vi "pp3_DAQ_AudioTriggerPlay.vi"(0 "Daq config In":T6={"Sound AO"="Dev2/ao0", "Shock intesity AO"="Dev1/ao1", "Code_LED DO"="Dev1/port1:2", "Switch DI"="Dev1/port0/line0:1", "Webcam"="cam0", "Sound AO task"="", "Sound card task"=0, "Shock intensity AO task"="", "Code_LED DO task"="", "Switch DI task"="", "AO <=> Sound card"=FALSE, "Sound card"=0, "sample rate"=8000.0, "Variable shock"=FALSE, "Webcam on"=FALSE, "Tone gate PFI"="/Dev1/PFI1", "Waveform memo"={"t0"=timestamp(0 s since 1904-01-01), "dt"=1.0, "Y"=[]}, "First time"=FALSE} {"sample rate" min=8000.0; "Sound card task" format="%.0x"}, 5 "State In":T1={"Curr  tr"=0, "Curr (ms)"=0, "Cum (ms)"=0, "Run loop diff"=0, "Tone countdown (ms)"=0, "Countdown (ms)"=0, "Curr State"=enum."0 NULL", "Prev State"=enum."1 Habituation", "Rw"=FALSE, "Sw"=FALSE, "Tone\nGate"=FALSE, "Punish"=FALSE, "Current DAQ DO Int"=0, "Current Loaded Trial"={"Trial Type Number"=1, "Trial Type"=enum."GO", "Trial Weight"=100, "Shock (mA)"=0.3, "Duration (ms)"=0.25, "Sound Type"=enum."04 FM Sweep", "Stim P1"=4000.0, "Stim P2"=0.0, "Stim P3"=0.0, "Stim P4"=2000.0, "DAQ Amplitude (V)"=0.25}, "Next Trial (for display purposes)"={"Trial Type Number"=1, "Trial Type"=enum."GO", "Trial Weight"=100, "Shock (mA)"=0.3, "Duration (ms)"=0.25, "Sound Type"=enum."04 FM Sweep", "Stim P1"=4000.0, "Stim P2"=0.0, "Stim P3"=0.0, "Stim P4"=2000.0, "DAQ Amplitude (V)"=0.25}, "Total trials memo"=0, "State start cum memo (ms)"=0, "Last dur jump time memo (ms)"=0, "Last dur shock time memo (ms)"=0, "Tone repeat memo (ms)"=0, "Webcam on"=FALSE, "Webcam recording"=FALSE, "State update flag"=FALSE, "Last loaded shock voltage"=0.0, "Vid upd"=enum."0"} {"Current DAQ DO Int" format="%016b"; "Next Trial (for display purposes)"."DAQ Amplitude (V)" min=0.0 max=5.0 format="%_6g"; "Next Trial (for display purposes)"."Shock (mA)" min=-1.0 max=5.0; "Next Trial (for display purposes)"."Trial Weight" step=1; "Next Trial (for display purposes)"."Duration (ms)" min=0.0 max=1.0; "Next Trial (for display purposes)"."Trial Type Number" min=1 max=256 step=1; "Current Loaded Trial"."DAQ Amplitude (V)" min=0.0 max=5.0 format="%_6g"; "Current Loaded Trial"."Shock (mA)" min=-1.0 max=5.0; "Current Loaded Trial"."Trial Weight" step=1; "Current Loaded Trial"."Duration (ms)" min=0.0 max=1.0; "Current Loaded Trial"."Trial Type Number" min=1 max=256 step=1}, 11 "error in (no error)":errorcluster) -> (4 "Daq config Out":T6={"Sound AO"="Dev2/ao0", "Shock intesity AO"="Dev1/ao1", "Code_LED DO"="Dev1/port1:2", "Switch DI"="Dev1/port0/line0:1", "Webcam"="cam0", "Sound AO task"="", "Sound card task"=0, "Shock intensity AO task"="", "Code_LED DO task"="", "Switch DI task"="", "AO <=> Sound card"=FALSE, "Sound card"=0, "sample rate"=8000.0, "Variable shock"=FALSE, "Webcam on"=FALSE, "Tone gate PFI"="/Dev1/PFI1", "Waveform memo"={"t0"=timestamp(0 s since 1904-01-01), "dt"=1.0, "Y"=[]}, "First time"=FALSE} {"sample rate" min=8000.0; "Sound card task" format="%.0x"}, 6 "State Out":T1={"Curr  tr"=0, "Curr (ms)"=0, "Cum (ms)"=0, "Run loop diff"=0, "Tone countdown (ms)"=0, "Countdown (ms)"=0, "Curr State"=enum."0 NULL", "Prev State"=enum."1 Habituation", "Rw"=FALSE, "Sw"=FALSE, "Tone\nGate"=FALSE, "Punish"=FALSE, "Current DAQ DO Int"=0, "Current Loaded Trial"={"Trial Type Number"=1, "Trial Type"=enum."GO", "Trial Weight"=100, "Shock (mA)"=0.3, "Duration (ms)"=0.25, "Sound Type"=enum."04 FM Sweep", "Stim P1"=4000.0, "Stim P2"=0.0, "Stim P3"=0.0, "Stim P4"=2000.0, "DAQ Amplitude (V)"=0.25}, "Next Trial (for display purposes)"={"Trial Type Number"=1, "Trial Type"=enum."GO", "Trial Weight"=100, "Shock (mA)"=0.3, "Duration (ms)"=0.25, "Sound Type"=enum."04 FM Sweep", "Stim P1"=4000.0, "Stim P2"=0.0, "Stim P3"=0.0, "Stim P4"=2000.0, "DAQ Amplitude (V)"=0.25}, "Total trials memo"=0, "State start cum memo (ms)"=0, "Last dur jump time memo (ms)"=0, "Last dur shock time memo (ms)"=0, "Tone repeat memo (ms)"=0, "Webcam on"=FALSE, "Webcam recording"=FALSE, "State update flag"=FALSE, "Last loaded shock voltage"=0.0, "Vid upd"=enum."0"} {"Current DAQ DO Int" format="%016b"; "Next Trial (for display purposes)"."DAQ Amplitude (V)" min=0.0 max=5.0 format="%_6g"; "Next Trial (for display purposes)"."Shock (mA)" min=-1.0 max=5.0; "Next Trial (for display purposes)"."Trial Weight" step=1; "Next Trial (for display purposes)"."Duration (ms)" min=0.0 max=1.0; "Next Trial (for display purposes)"."Trial Type Number" min=1 max=256 step=1; "Current Loaded Trial"."DAQ Amplitude (V)" min=0.0 max=5.0 format="%_6g"; "Current Loaded Trial"."Shock (mA)" min=-1.0 max=5.0; "Current Loaded Trial"."Trial Weight" step=1; "Current Loaded Trial"."Duration (ms)" min=0.0 max=1.0; "Current Loaded Trial"."Trial Type Number" min=1 max=256 step=1}, 15 "error out":errorcluster)   [LabVIEW 2013]
uses:
  pp2_CTL_DaqConfig.ctl
  <vilib>/userdefined/High Color/IMAQdx.ctl
  <vilib>/sound2/lvsound2.llb/Sound Output Task ID.ctl
  pp3_CTL_StateInfo.ctl
  pp3_CTL_State.ctl
  pp3_CTL_Trial.ctl
  pp3_CTL_TrialType.ctl
  labolabo2/waveforms/WFTypes.ctl
  <vilib>/sound2/lvsound2.llb/Sound Output Write (DBL Single).vi
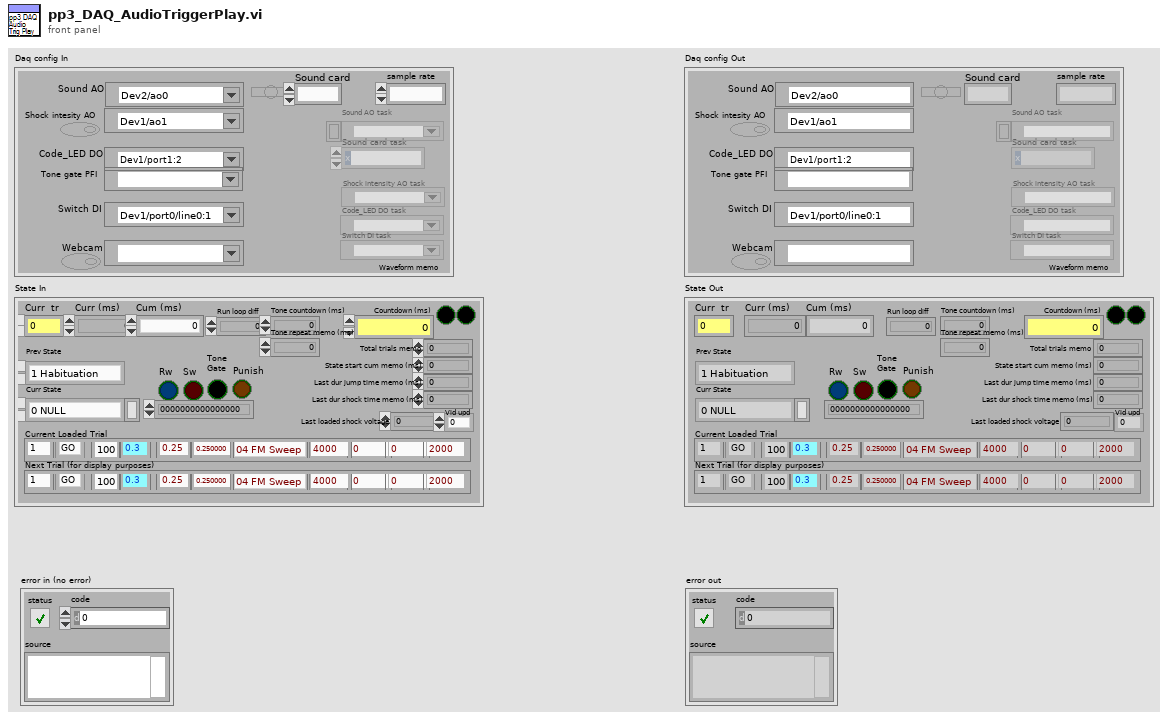
[diagram p1: front panel]
types:
  T1 = typedef "pp3_CTL_StateInfo.ctl" = cluster{"Curr  tr":u16, "Curr (ms)":u32, "Cum (ms)":i64, "Run loop diff":i64, "Tone countdown (ms)":i64, "Countdown (ms)":i64, "Curr State":T2, "Prev State":T2, "Rw":bool, "Sw":bool, "Tone\nGate":bool, "Punish":bool, "Current DAQ DO Int":u16, "Current Loaded Trial":T3, "Next Trial (for display purposes)":T3, "Total trials memo":i64, "State start cum memo (ms)":i64, "Last dur jump time memo (ms)":i64, "Last dur shock time memo (ms)":i64, "Tone repeat memo (ms)":i64, "Webcam on":bool, "Webcam recording":bool, "State update flag":bool, "Last loaded shock voltage":dbl, "Vid upd":enum16{"0", "1", "2", "3", "4", "5", "6", "7", "8", "9"}}
  T2 = typedef "pp3_CTL_State.ctl" = enum8{"0 NULL", "1 Habituation", "2 (Load Trial)", "3 Stay Period", "4 Load Audio/Click Delay", "5 GO Trial", "6 GO Jumped", "7 GO Timeout", "8 NOGO Trial", "9 NOGO Jumped", "10 NOGO Timeout", "11 TEST Trial", "12 TEST Jumped", "13 TEST Timeout", "14 Intertrial Interval", "15 Done"}
  T3 = typedef "pp3_CTL_Trial.ctl" = cluster{"Trial Type Number":i16, "Trial Type":T4, "Trial Weight":u32, "Shock (mA)":dbl, "Duration (ms)":dbl, "Sound Type":T5, "Stim P1":dbl, "Stim P2":dbl, "Stim P3":dbl, "Stim P4":dbl, "DAQ Amplitude (V)":dbl}
  T4 = typedef "pp3_CTL_TrialType.ctl" = enum16{"OFF", "GO", "NOGO", "TEST"}
  T5 = typedef "WFTypes.ctl" = enum16{"00 NULL", "01 DC", "02 Noise", "03 Pure Tone", "04 FM Sweep"}
  T6 = typedef "pp2_CTL_DaqConfig.ctl" = cluster{"Sound AO":tag, "Shock intesity AO":tag, "Code_LED DO":tag, "Switch DI":tag, "Webcam":T7, "Sound AO task":refnum<k21>, "Sound card task":T8, "Shock intensity AO task":refnum<k21>, "Code_LED DO task":refnum<k21>, "Switch DI task":refnum<k21>, "AO <=> Sound card":bool, "Sound card":u32, "sample rate":dbl, "Variable shock":bool, "Webcam on":bool, "Tone gate PFI":tag, "Waveform memo":waveform(dbl), "First time":bool}
  T7 = typedef "IMAQdx.ctl" = refnum<k21>
  T8 = typedef "Sound Output Task ID.ctl" = u32
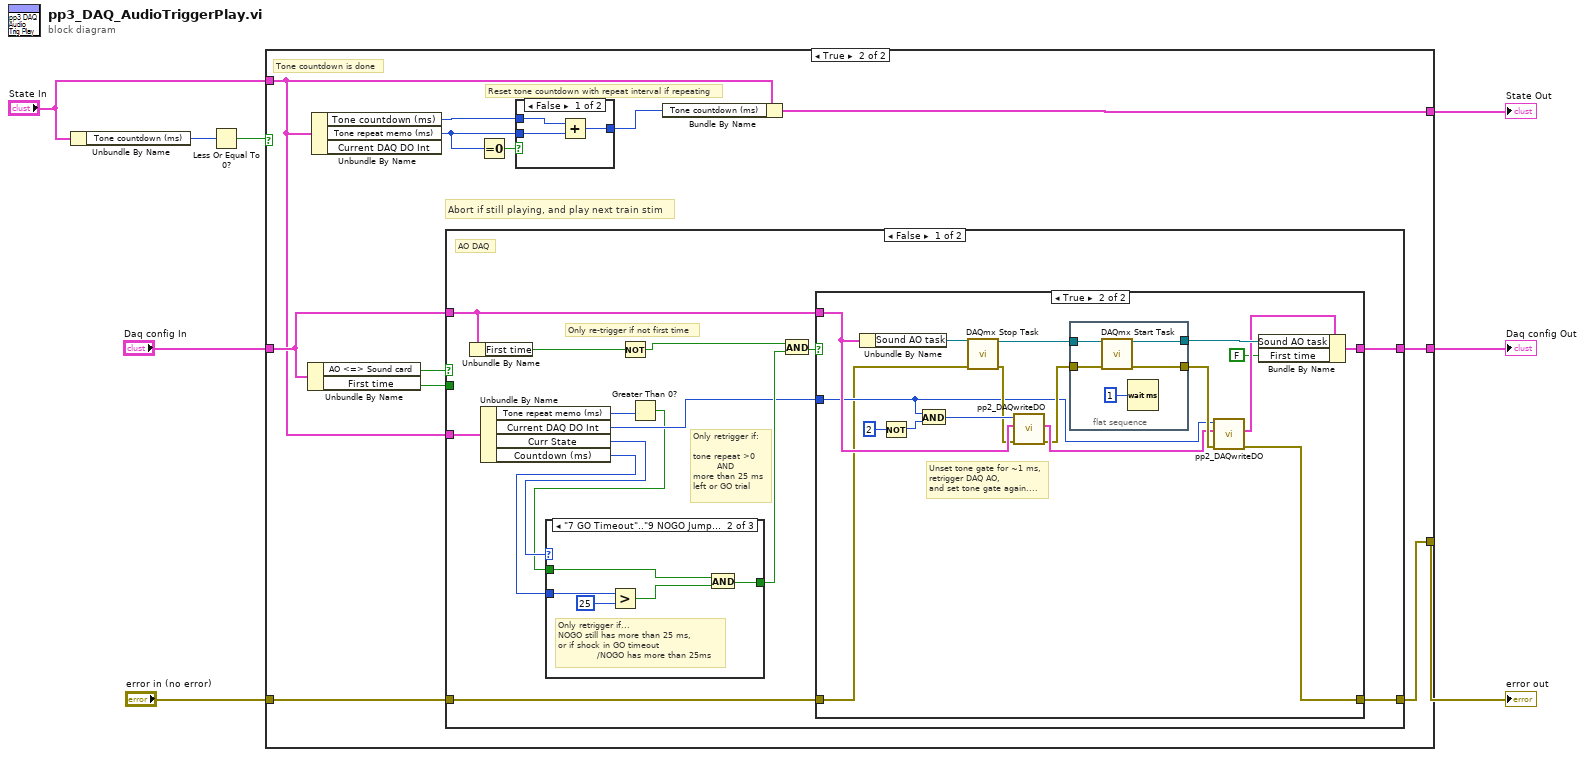
[diagram p0: block diagram]
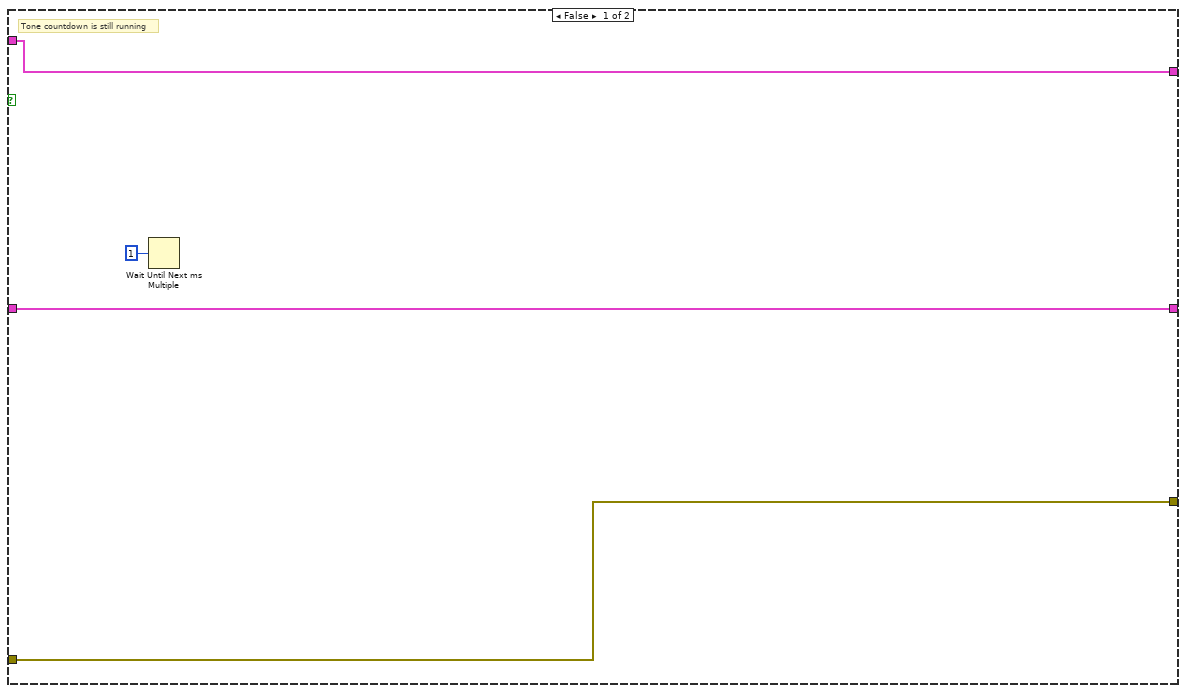
[diagram p2: hidden frame]
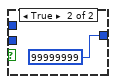
[diagram p3: hidden frame]
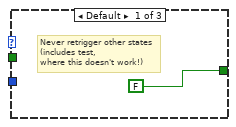
[diagram p4: hidden frame]
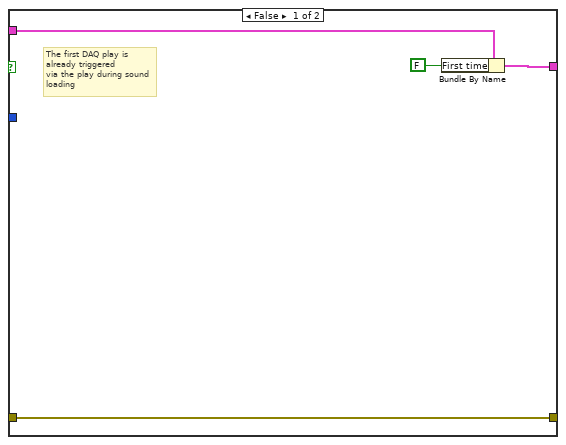
[diagram p6: hidden frame]
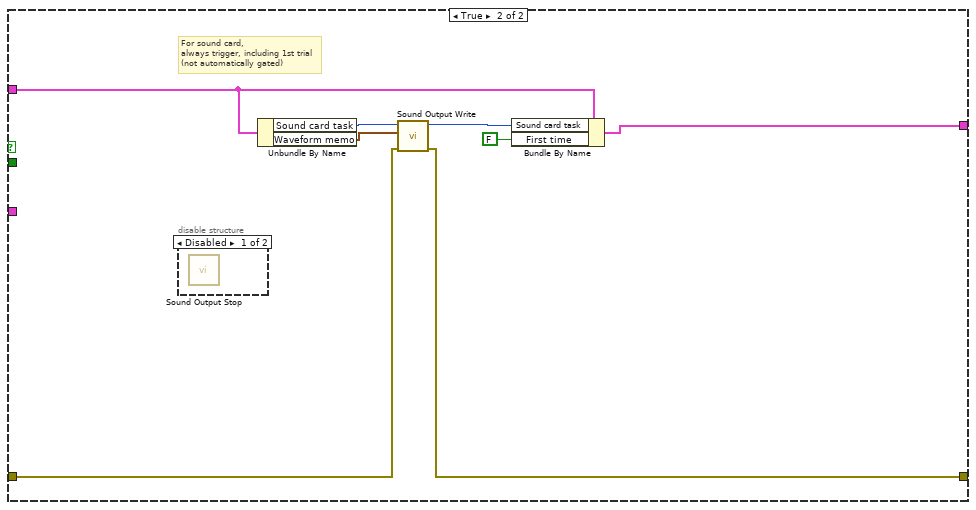
[diagram p7: hidden frame]
diagram:
  n1 = Unbundle By Name("State In") -> ("Tone countdown (ms)"=w4:i64)
  n2 = Less Or Equal To 0?(x=w4) -> (x <= 0?=w1:bool)
  n3 = case shown="True" w1 {
    tunnel: "Daq config In" -> [w12 w21]
    tunnel: [w12 w20] -> w7
    tunnel: "error in (no error)" -> [w11 w23]
    tunnel: [w11 w22] -> w5
    tunnel: "State In" -> [w9 w13]
    tunnel: [w9 w19] -> w2
    frame False {
      # "Tone countdown is still running"
      n4 = Wait Until Next ms Multiple(millisecond multiple=u32 1) -> ()  [unwired: 1 out]
    }
    frame True {
      # "Tone countdown is done"
      # "Abort if still playing, and play next train stim"
      # "Reset tone countdown with repeat interval if repeating"
      n5 = Unbundle By Name(w21) -> ("AO <=> Sound card"=w24:bool, "First time"=w18:bool)
      n6 = Unbundle By Name(w13) -> ("Tone countdown (ms)"=w15:i64, "Tone repeat memo (ms)"=w16:i64)  [unwired: 1 out]
      n7 = case shown="False" w24 {
        tunnel: w23 -> [w34 w83]
        tunnel: [w42 w82] -> w22
        tunnel: w21 -> [w41 w80]
        tunnel: [w40 w81] -> w20
        tunnel: w18 -> [_ _]
        tunnel: w13 -> [w39 _]
        frame False {
          # "Only retrigger if:\n\ntone repeat >0\n        AND\nmore than 25 ms\nleft or GO trial"
          # "Only re-trigger if not first time"
          # "AO DAQ"
          n8 = Unbundle By Name(w41) -> ("First time"=w38:bool)
          n9 = Unbundle By Name(w39) -> ("Tone repeat memo (ms)"=w30:i64, "Current DAQ DO Int"=w31:u16, "Curr State"=w33:T2, "Countdown (ms)"=w32:i64)
          n10 = Not(x=w38) -> (.not. x?=w36:bool)
          n11 = Greater Than 0?(x=w30) -> (x > 0?=w29:bool)
          n12 = case shown="\"7 GO Timeout\"..\"9 NOGO Jumped\"" w33 {
            tunnel: [FALSE w46 w49] -> w35
            tunnel: w32 -> [_ w47 _]
            tunnel: w29 -> [_ w44 w49]
            frame Default {
              # "Never retrigger other states\n(includes test, \nwhere this doesn't work!)"
            }
            frame "7 GO Timeout".."9 NOGO Jumped" {
              # "Only retrigger if...\nNOGO still has more than 25 ms, \nor if shock in GO timeout\n             /NOGO has more than 25ms"
              n13 = Greater?(x=w47, y=i64 25) -> (0:w45:bool)
              n14 = And(x=w44, y=w45) -> (x .and. y?=w46:bool)
            }
            frame "5 GO Trial" {
              # "GO Trial will always be retriggered\nwhen done,\nsince ending will lead to\ntone continuation and shock"
            }
          }
          n15 = And(x=w36, y=w35) -> (x .and. y?=w37:bool)
          n16 = case shown="True" w37 {
            tunnel: w34 -> [w53 w55]
            tunnel: [w53 w62] -> w42
            tunnel: w41 -> [w51 w61]
            tunnel: [w50 w67] -> w40
            tunnel: w31 -> [_ w56]
            frame False {
              # "The first DAQ play is\nalready triggered\nvia the play during sound\nloading"
              n17 = Bundle By Name(cluster=w51, "First time"=FALSE) -> (w50:T6)
            }
            frame True {
              # "Unset tone gate for ~1 ms,\nretrigger DAQ AO,\nand set tone gate again...."
              n18 = Unbundle By Name(w61) -> ("Sound AO task"=w68:refnum<k21>)
              n19 = Not(x=u16 2) -> (.not. x?=w65:u16)
              n20 = And(x=w56, y=w65) -> (x .and. y?=w64:u16)
              n21 = call <vilib>:"DAQmx Stop Task.vi"("task/channels in"=w68, "error in"=w55) -> ("task out"=w70:refnum<k21>, "error out"=w58:errorcluster)  [unwired: 12 in]
              n22 = call "pp2_DAQwriteDO.vi"("error in (no error)"=w58, "Daq config"=w61, "DAQ Digital In"=w64) -> ("error out"=w57:errorcluster, "Daq config 2"=w60:T6)  [unwired: 7 in]
              n23 = flat-sequence {
                tunnel: w70 -> [w75]
                tunnel: [w74] -> w63
                tunnel: [w73] -> w69
                tunnel: w57 -> [w71]
                frame #0 {
                  n24 = call <vilib>:"DAQmx Start Task.vi"("task/channels in"=w75, "error in"=w71) -> ("task out"=w73:refnum<k21>, "error out"=w74:errorcluster)  [unwired: 12 in]
                  n25 = Wait (ms)(milliseconds to wait=u32 1) -> ()  [unwired: 1 out]
                }
              }
              n26 = call "pp2_DAQwriteDO.vi"("error in (no error)"=w63, "Daq config"=w60, "DAQ Digital In"=w56) -> ("error out"=w62:errorcluster, "Daq config 2"=w59:T6)  [unwired: 7 in]
              n27 = Bundle By Name(cluster=w59, "Sound AO task"=w69, "First time"=FALSE) -> (w67:T6)
            }
          }
        }
        frame True {
          # "For sound card,\nalways trigger, including 1st trial\n(not automatically gated)"
          n28 = disable-structure shown="Disabled" {
            frame Disabled {
              n29 = call <vilib>:"Sound Output Stop.vi"() -> ()  [unwired: 10 in, 2 out]
            }
            frame Enabled {
            }
          }
          n30 = Unbundle By Name(w80) -> ("Sound card task"=w79:T8, "Waveform memo"=w78:waveform(dbl))
          n31 = call-poly <vilib>:"Sound Output Write.vi"("error in (no error)"=w83, "data"=w78, "task ID"=w79) -> ("error out"=w82:errorcluster, "task ID out"=w77:T8)  [unwired: 7 in]
          n32 = Bundle By Name(cluster=w80, "Sound card task"=w77, "First time"=FALSE) -> (w81:T6)
        }
      }
      n33 = Equal To 0?(x=w16) -> (x = 0?=w17:bool)
      n34 = case shown="False" w17 {
        tunnel: w16 -> [w26 _]
        tunnel: w15 -> [w27 _]
        tunnel: [w25 i64 99999999] -> w14
        frame False {
          n35 = Add(x=w27, y=w26) -> (x+y=w25:i64)
        }
        frame True {
        }
      }
      n36 = Bundle By Name(cluster=w13, "Tone countdown (ms)"=w14) -> (w19:T1)
    }
  }
  "Daq config Out" <- w7
  "error out" <- w5
  "State Out" <- w2
